vi "UDP Map Tag to Last Update Channel.vi"(8 "error in (no error)":errorcluster, 10 "Tag Name":string, 11 "node References":T1) -> (0 "error out":errorcluster, 3 "node References out":T1)   [LabVIEW 2015, in "E2E Tag Exchange editor node.lvclass"]
uses:
  E2E Tag Exchange editor node.lvclass
  object references.ctl
  <vilib>/NI/DCAF/Tag Editor Core/Configuration Editor/Classes/Engine Parent/Engine Parent Editor Node.lvclass
  <vilib>/NI/Module Execution Interface/Engine Configuration/engine configuration.lvclass
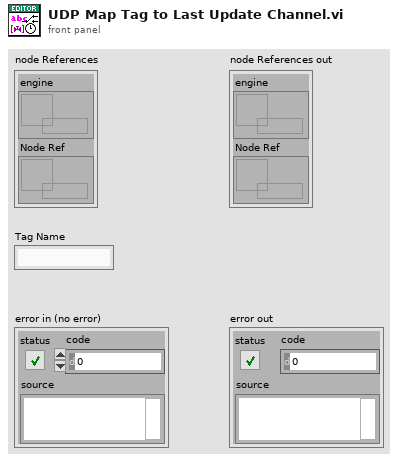
[diagram p1: front panel]
types:
  T1 = typedef "E2E Tag Exchange editor node.lvclass/object references.ctl" = cluster{"engine":refnum<data-value>, "Node Ref":refnum<data-value>}
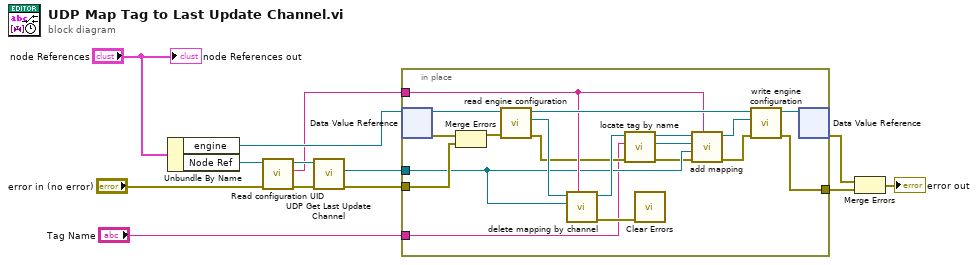
[diagram p0: block diagram]
diagram:
  n1 = Unbundle By Name("node References") -> ("engine"=w11:refnum<data-value>, "Node Ref"=w9:refnum<data-value>)
  n2 = call "Read configuration UID.vi"("error in (no error)"="error in (no error)", "E2E editor node in"=w9) -> ("error out"=w7:errorcluster, "Module UID"=w6:string, "E2E editor node out"=w8:refnum<data-value>)  [unwired: 7 in]
  n3 = call "UDP Get Last Update Channel.vi"("error in (no error)"=w7, "E2E editor node in"=w8) -> ("error out"=w5:errorcluster, "channel out"=w12:refnum<class "TBM channel.lvclass">)  [unwired: 7 in, 1 out]
  n4 = in-place {
    in-place-border: w12 -> [w16]
    in-place-border: "Tag Name" -> [w14]
    in-place-border: w6 -> [w22]
    in-place-border: w5 -> [w27]
    in-place-border: [w24] -> w3
    n5 = in-place-dvr #1(w11) -> (w32:refnum<class "Engine Parent Editor Node.lvclass">, w26:errorcluster)
    n6 = Merge Errors(w26, w27) -> (w25:errorcluster)
    n7 = call <vilib>:"read engine configuration.vi"("error in"=w25, "Engine Parent Editor Node in"=w32) -> ("error out"=w20:errorcluster, "engine configuration"=w23:refnum<class "engine configuration.lvclass">, "Engine Parent Editor Node out"=w31:refnum<class "Engine Parent Editor Node.lvclass">)  [unwired: 7 in]
    n8 = call <vilib>:"delete mapping by channel.vi"("owner ID"=w22, "channel"=w16, "engine configuration in"=w23) -> ("error out"=w17:errorcluster, "engine configuration out"=w21:refnum<class "engine configuration.lvclass">)  [unwired: 7 in]
    n9 = call <vilib>:"locate tag by name.vi"("error in"=w20, "tag name"=w14, "engine configuration in"=w21) -> ("error out"=w15:errorcluster, "tag descriptor"=w19:refnum<class "tag descriptor.lvclass">, "engine configuration out"=w18:refnum<class "engine configuration.lvclass">)  [unwired: 6 in]
    n10 = call <vilib>:"Clear Errors.vi"("error in (no error)"=w17) -> ()  [unwired: 5 in, 2 out]
    n11 = call-dynamic "add mapping.vi"("owner ID"=w22, "error in"=w15, "channel"=w16, "tag descriptor"=w19, "engine configuration"=w18) -> ("error out"=w29:errorcluster, "engine configuration out"=w28:refnum<class "engine configuration.lvclass">)  [unwired: 5 in]
    n12 = call <vilib>:"write engine configuration.vi"("error in"=w29, "engine configuration"=w28, "Engine Parent Editor Node in"=w31) -> ("error out"=w24:errorcluster, "Engine Parent Editor Node out"=w30:refnum<class "Engine Parent Editor Node.lvclass">)  [unwired: 7 in]
    n13 = in-place-dvr #1(w30) -> (w2:errorcluster)  [unwired: 1 out]
  }
  n14 = Merge Errors(w2, w3) -> (→"error out":errorcluster)
  "node References out" <- "node References"
